vi "Create Layer.vi"() -> ()   [LabVIEW 2021, in "Galaxy.lvclass"]
uses:
  Galaxy.lvclass
panel:
  in  "Number Of Textures":dbl
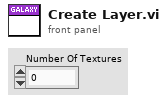
[diagram p1: front panel]
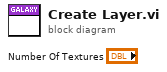
[diagram p0: block diagram]
diagram:
